vi "Read Distance Data.vi"(11 "DistanceGauge in":refnum<class "DistanceGauge.lvclass">) -> (2 "Distance Data":T1={"Distance Measured 1"=1.0, "Distance Measured 2"=1.0} {"Distance Measured 2" min=1.0 max=300.0 format="%.1f"; "Distance Measured 1" min=1.0 max=300.0 format="%.1f"}, 3 "DistanceGauge out":refnum<class "DistanceGauge.lvclass">)   [LabVIEW 2013, in "DistanceGauge.lvclass"]
uses:
  DistanceGauge.lvclass
  Typedefs/Distance Data.ctl
  DistanceGauge.lvclass/DistanceGauge.ctl
  Typedefs/M2AADTTypedefs.lvlib
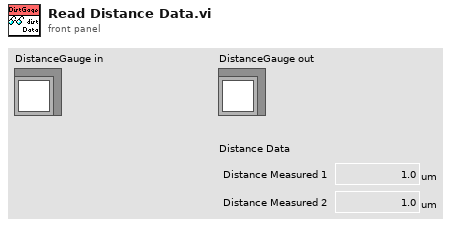
[diagram p1: front panel]
types:
  T1 = typedef "M2AADTTypedefs.lvlib/Distance Data.ctl" = cluster{"Distance Measured 1":dbl[unit], "Distance Measured 2":dbl[unit]}
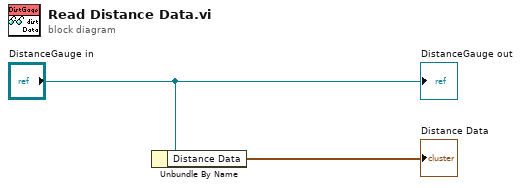
[diagram p0: block diagram]
diagram:
  n1 = Unbundle By Name("DistanceGauge in") -> ("Distance Data"=→"Distance Data":T1)
  "DistanceGauge out" <- "DistanceGauge in"
